vi "Convert Res. to Temp..vi"(6 "error in":errorcluster, 8 "Convert to Temp.":bool, 9 "Calibration FIle":path, 10 "Channel":string, 11 "Y Array":dbl[](array[numeric])) -> (3 "Y Array":dbl[](array[numeric]), 4 "error out":errorcluster)   [LabVIEW 2023]
uses:
  <vilib>/Utility/file.llb/Read Delimited Spreadsheet (string).vi
  <vilib>/Utility/file.llb/Read Delimited Spreadsheet (DBL).vi
  <vilib>/gmath/NI_Gmath.lvlib
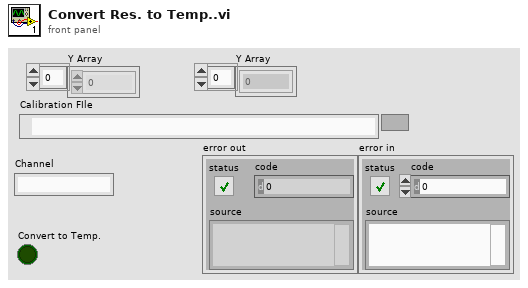
[diagram p1: front panel]
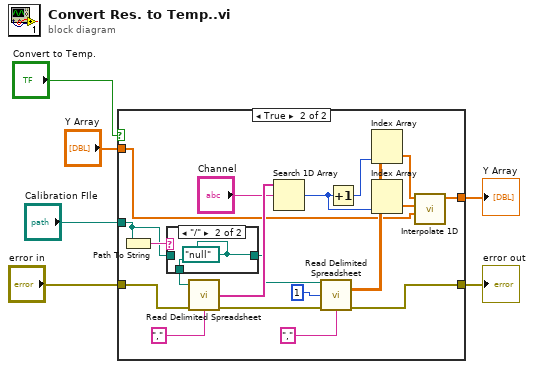
[diagram p0: block diagram]
diagram:
  n1 = case shown="True" "Convert to Temp." {
    tunnel: "Calibration FIle" -> [_ w11]
    tunnel: "Y Array" -> [w8 w17]
    tunnel: [w8 w16] -> w4
    tunnel: [w7 w14] -> w2
    tunnel: "error in" -> [w7 w13]
    frame False {
    }
    frame True {
      n2 = Path To String(path=w11) -> (string=w12:string)
      n3 = case shown="\"/\"" w12 {
        tunnel: w11 -> [w28 _]
        tunnel: [w28 w29] -> w9
        tunnel: [w28 w29] -> w10
        frame Default {
        }
        frame "/" {
          w29 = path "/null" ("Calibration FIle")
        }
      }
      n4 = call-poly <vilib>:"Read Delimited Spreadsheet.vi"("file path (dialog if empty)"=w9, "error in (no error)"=w13, "delimiter (\\t)"=",") -> ("first row"=w26:string[], "error out"=w15:errorcluster)  [unwired: 7 in, 4 out]
      n5 = Search 1D Array(1D array=w26, element="Channel") -> (index of element=w22:i32)  [unwired: 1 in]
      n6 = call-poly <vilib>:"Read Delimited Spreadsheet.vi"("file path (dialog if empty)"=w10, "start of read offset (chars.:0)"=1, "error in (no error)"=w15, "delimiter (\\t)"=",") -> ("all rows"=w19:dbl[][], "error out"=w14:errorcluster)  [unwired: 6 in, 4 out]
      n7 = Increment(x=w22) -> (x+1=w21:i32)
      n8 = Index Array(array=w19, index (col)=w21) -> (element=w18:dbl[])  [unwired: 1 in]
      n9 = Index Array(array=w19, index (col)=w22) -> (element=w20:dbl[])  [unwired: 1 in]
      n10 = call <vilib>:"Interpolate 1D.vi"("xi"=w17, "X"=w20, "Y"=w18) -> ("yi"=w16:dbl[])  [unwired: 6 in, 2 out]
    }
  }
  "Y Array" <- w4
  "error out" <- w2
